vi "Event Queue Self Alias.vi"(11 "Hello World Event in":refnum<class "Hello World Event.lvclass">) -> (2 "Queue Self Alias":string, 3 "Hello World Event out":refnum<class "Hello World Event.lvclass">)   [LabVIEW 2021, in "Hello World Event.lvlib" / "Hello World Event.lvclass"]
uses:
  Hello World Event.lvclass
  Hello World Event.lvclass/Hello World Event.ctl
  jettl/Event jettl/Event jettl.lvclass
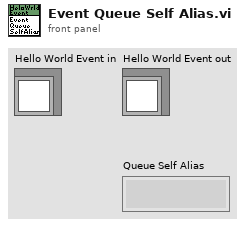
[diagram p1: front panel]
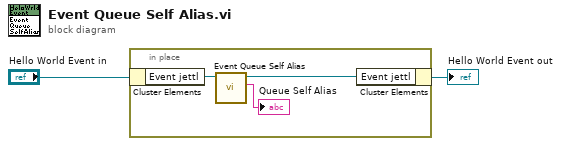
[diagram p0: block diagram]
diagram:
  n1 = in-place {
    n2 = in-place-cluster #1("Hello World Event in") -> ("Event jettl"=w5:refnum<class "Event jettl.lvclass">)
    n3 = call-dynamic "Event Queue Self Alias.vi"("Event jettl in"=w5) -> ("Queue Self Alias"=→"Queue Self Alias":string, "Event jettl out"=w4:refnum<class "Event jettl.lvclass">)  [unwired: 9 in]
    n4 = in-place-cluster #1("Event jettl"=w4) -> (→"Hello World Event out":refnum<class "Hello World Event.lvclass">)
  }
